vi "QuantizeFloat32.vi"(7 "sticky bit":bool, 10 "float in":T1 {"mantissa" format="%08x"}) -> (3 "float out":T1 {"mantissa" format="%08x"})   [LabVIEW 2011]
uses:
  FPGA SGL.ctl
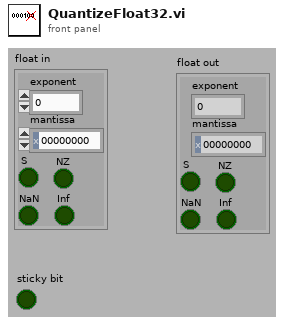
[diagram p1: front panel]
types:
  T1 = typedef "FPGA SGL.ctl" = cluster{"exponent":u8, "mantissa":u32, "S":bool, "NZ":bool, "NaN":bool, "Inf":bool}
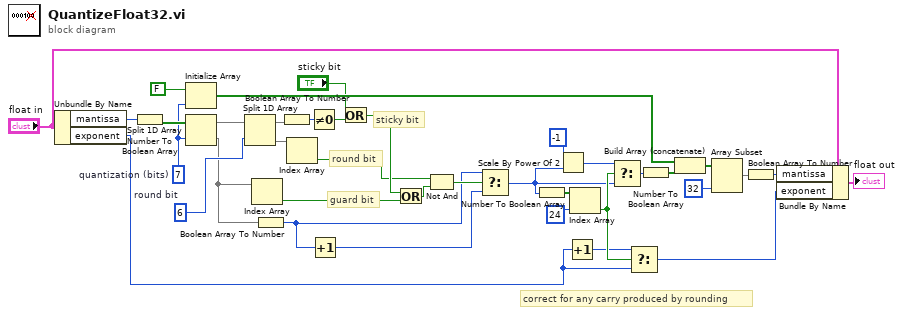
[diagram p0: block diagram]
diagram:
  w22 = 6  # round bit
  w23 = i8 7  # quantization (bits)
  # "correct for any carry produced by rounding"
  # "guard bit"
  # "round bit"
  # "sticky bit"
  n1 = Unbundle By Name("float in") -> ("mantissa"=w35:u32, "exponent"=w11:u8)
  n2 = Number To Boolean Array(number=w35) -> (Boolean array=w33:bool[])
  n3 = Initialize Array(FALSE, w23) -> (w27:bool[])
  n4 = Split 1D Array(array=w33, index=w23) -> (first subarray=w32:bool[], second subarray=w9:bool[])
  n5 = Split 1D Array(array=w32, index=w22) -> (first subarray=w31:bool[], second subarray=w29:bool[])
  n6 = Index Array(array=w9) -> (element=w6:bool)  [unwired: 1 in]
  n7 = Boolean Array To Number(Boolean array=w9) -> (number=w3:u32)
  n8 = Boolean Array To Number(Boolean array=w31) -> (number=w30:u8)
  n9 = Index Array(array=w29) -> (element=w4:bool)  [unwired: 1 in]
  n10 = Not Equal To 0?(x=w30) -> (x != 0?=w21:bool)
  n11 = Increment(x=w3) -> (x+1=w2:u32)
  n12 = Or(x="sticky bit", y=w21) -> (x .or. y?=w5:bool)
  n13 = Or(x=w5, y=w6) -> (x .or. y?=w7:bool)
  n14 = Not And(1:w7, 2:w4) -> (0:w8:bool)
  n15 = Select(t=w3, s=w8, f=w2) -> (s? t:f=w1:u32)
  n16 = Number To Boolean Array(number=w1) -> (Boolean array=w19:bool[])
  n17 = Scale By Power Of 2(n=-1, x=w1) -> (x*2^n=w16:u32)
  n18 = Increment(x=w11) -> (x+1=w12:u8)
  n19 = Index Array(array=w19, index=24) -> (element=w13:bool)
  n20 = Select(t=w16, s=w13, f=w1) -> (s? t:f=w15:u32)
  n21 = Select(t=w12, s=w13, f=w11) -> (s? t:f=w10:u8)
  n22 = Number To Boolean Array(number=w15) -> (Boolean array=w14:bool[])
  n23 = Build Array (concatenate)(w27, w14) -> (w25:bool[])
  n24 = Array Subset(array=w25, length=32) -> (w26:bool[])  [unwired: 1 in]
  n25 = Boolean Array To Number(Boolean array=w26) -> (number=w34:u32)
  n26 = Bundle By Name(cluster="float in", "mantissa"=w34, "exponent"=w10) -> (→"float out":T1)
